vi "rotary_PKP214_stiffness_test.vi"() -> ()   [LabVIEW 2014]
uses:
  <vilib>/rvi/FXPMathLib/FxpSinAndCos/subVIs/nifxpmath_SinAndCos_SimConfig.ctl
  <vilib>/rvi/Emulation/niFpgaGetClockAttributes.vi
  <vilib>/rvi/Emulation/niFpgaSctlEmulationGetInTimedLoop.vi
  <vilib>/rvi/Emulation/niFpgaEmulationReportErrorSimple.vi
  <vilib>/rvi/eio/common/nirviEmuTemplateMethod_errors.vi
  <vilib>/rvi/Emulation/niFpgaProcessEmulError.vi
  <vilib>/rvi/Emulation/niFpgaCriticalErrorInLSC.vi
  <vilib>/rvi/FXPMathLib/FxpSinAndCos/simVIs/DllFxpSinAndCosTemp_sub.vi
  <vilib>/rvi/interface/RandomDataEmulation/nirviRandomDataMultiElementFPGAFIFO.vi
  <instcachedir>/0/nirviRandomDataMultiElementFPGAFIFO_AD0CFC12EF974623A9C2E4184BC062B2.lvgen/nirviRandomDataMultiElementFPGAFIFO_AD0CFC12EF974623A9C2E4184BC062B2_023.vi
  <vilib>/rvi/interface/RandomDataEmulation/niFpgaRandomDataHandleErrors.vi
  <vilib>/eio/EIONode/EIONode.xnode
  <vilib>/rvi/FXPMathLib/FxpMul/XNode/nifxpmath_Multiplier.xnode
  <vilib>/rvi/FXPMathLib/FxpSinAndCos/XNode/nifxpmath_SinAndCos.xnode
  <vilib>/rvi/Analysis/measure/butterworth/XNode/niFpgaButterworthFilter.xnode
  <vilib>/rvi/FXPMathLib/FxpSub/XNode/nifxpmath_Sub.xnode
  <vilib>/rvi/FXPMathLib/FxpAdd/XNode/nifxpmath_Add.xnode
  <vilib>/rvi/DataTransferAndStorage/Container/XNode/niFpgaContainer.xnode
  <vilib>/rvi/interface/RandomDataEmulation/nirviRandomDataFpgaMultiElementTemplate.vi
  <vilib>/rvi/FXPMathLib/sim/FxpSim.dll
panel:
  out "Thetamr_dd":fxp<+/-,36,29>
  in  "thetam_limit (rad)":fxp<+/-,22,8>
  in  "Load cell start":bool
  in  "Load cell stop":bool
  in  "Load cell reset":bool
  out "Load cell 0":fxp<+/-,60,14>
  out "Load cell 1":fxp<+/-,60,14>
  in  "Magnetic Encoder Reset":bool
  out "Magnetic Encoder Position":i32
  out "Theta_a":fxp<+/-,33,18>
  out "Thetam":fxp<+/-,33,18>
  in  "Frequency_start (Hz)":fxp<+/-,22,8>
  in  "Target time (s)":fxp<+/-,24,9>
  in  "Frequency_end (Hz)":fxp<+/-,23,8>
  out "Chirp_signal":fxp<+/-,36,11>
  in  "Sin wave ampitude (rad)":fxp<+/-,21,11>
  out "omega (M_avg)":fxp<+/-,64,35>
  in  "D_d_M_avg_Tc (uSec)":u32
  out "omega (M)":fxp<+/-,64,30>
  in  "D_d_M_Tc (uSec)":u32 format="%#_6f"
  out "omega(T)":fxp<+/-,20,9>
  in  "Velocity Estimation":i16(ring) items=["M_avg method", "M method", "T method"]
  out "Thetamr_ramp":fxp<+/-,64,30>
  out "Thetamr_slope":fxp<+/-,33,17>
  in  "Thetamr_time":fxp<+/-,16,11>
  out "Thetamr_sin":fxp<+/-,28,11>
  out "Thetamr_sin_d":fxp<+/-,64,16>
  out "Thetamr_sin_dd":fxp<+/-,64,25>
  out "Sin omega":fxp<+/-,41,8>
  in  "Sin offset":fxp<+/-,27,10>
  in  "Sin magnitude":fxp<+/-,17,8>
  in  "Sin wave frequency (Hz)":fxp<+/-,21,5>
  out "Time now (s)":fxp<+,52,14>
  out "Thetamr":fxp<+/-,64,31>
  in  "Thetamr_end":fxp<+/-,19,9>
  in  "Command type":i16(ring) items=["Step", "Ramp", "Sine", "Chirp"]
  out "Thetam_i":fxp<+/-,34,18>
  in  "D_tolorence":fxp<+/-,14,3>
  in  "Ki":fxp<+/-,22,9>
  out "Thetam_error":fxp<+/-,24,11>
  in  "Direction":bool
  out "taur":fxp<+/-,64,31>
  in  "Kd":fxp<+/-,20,8>
  in  "Kp":fxp<+/-,20,12>
  in  "scaled coefficients_D_dd":i32[](array[numeric])=[780119100, 146811362]
  out "Thetam_dd":fxp<+/-,36,29>
  in  "Ini coe.":bool
  out "va":fxp<+/-,38,8>
  out "vb":fxp<+/-,38,8>
  in  "stop motor":bool
  out "vq_F":fxp<+/-,20,5> format="%.57g"
  out "vd_F":fxp<+/-,20,5>
  out "mt":u32
  out "omega (rad/s)":fxp<+/-,32,18>
  in  "mt0":u32
  out "NrTheta":fxp<+/-,33,18>
  out "Encoder Position":i32
  in  "Encoder Reset":bool
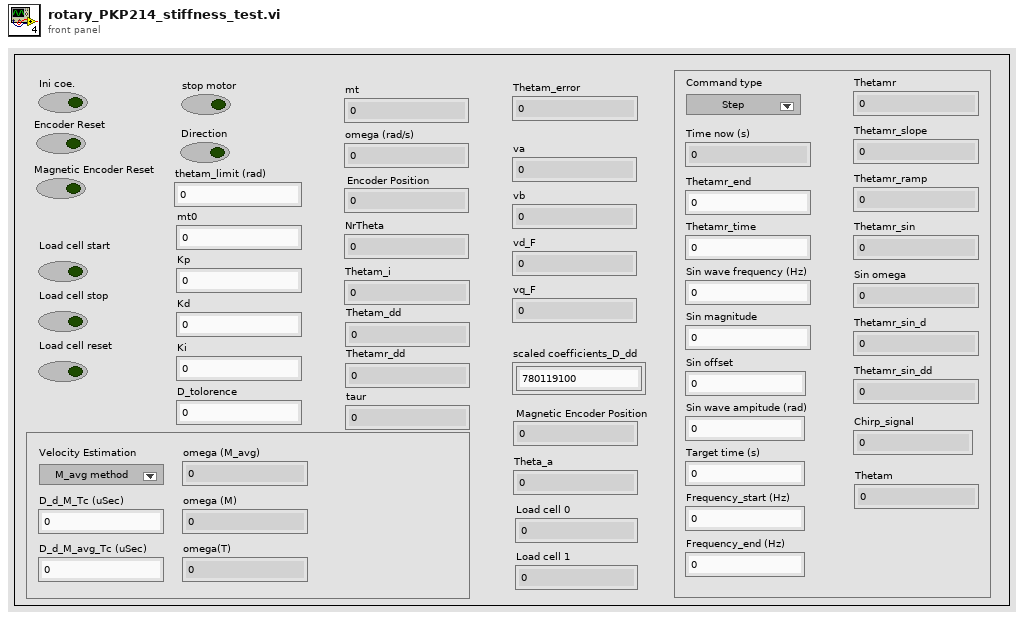
[diagram p1: front panel]
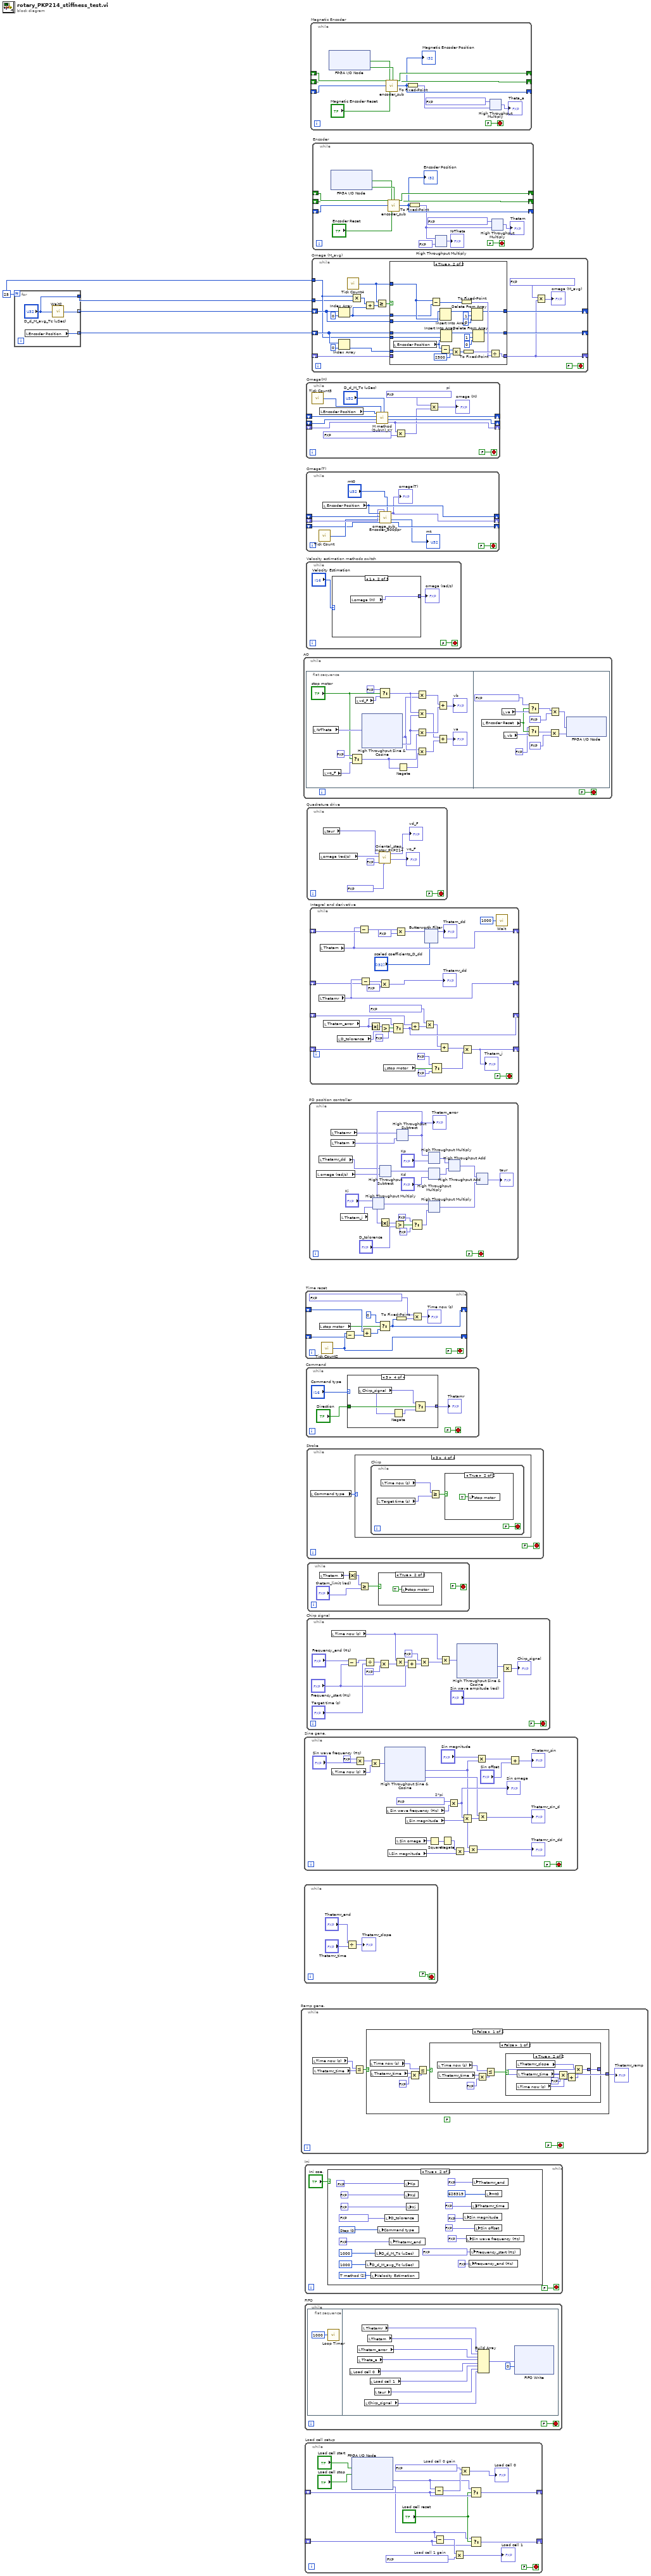
[diagram p0: block diagram]
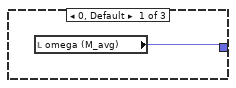
[diagram p4: hidden frame]
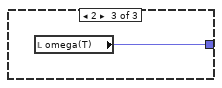
[diagram p5: hidden frame]
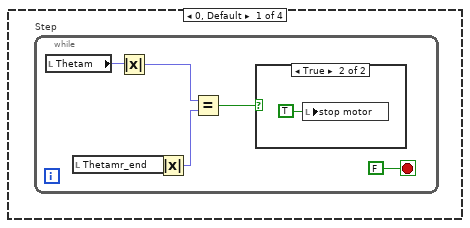
[diagram p6: hidden frame]
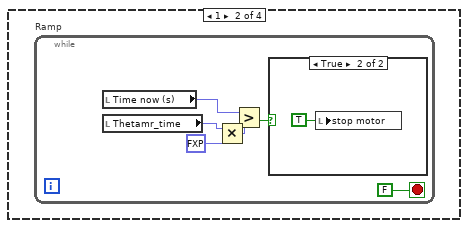
[diagram p8: hidden frame]
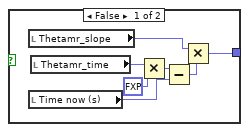
[diagram p12: hidden frame]
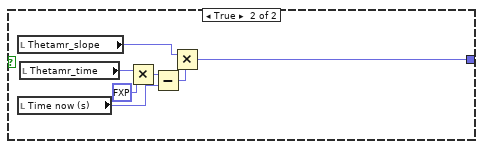
[diagram p13: hidden frame]
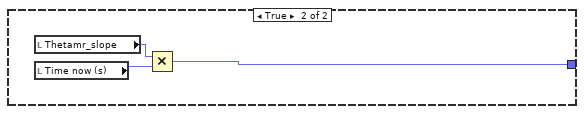
[diagram p14: hidden frame]
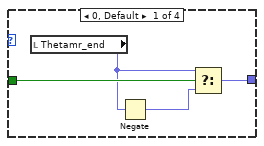
[diagram p15: hidden frame]
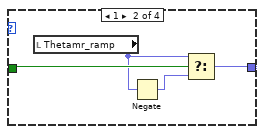
[diagram p16: hidden frame]
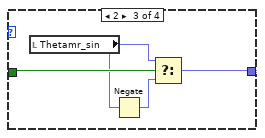
[diagram p17: hidden frame]
diagram:
  w4 = 25
  n1 = for {
    N: w4 -> [_]
    tunnel: ["D_d_M_avg_Tc (uSec)"] -> w1
    tunnel: [w6] -> w3 mode=indexing
    tunnel: [w5] -> w2 mode=indexing
    n2 = local read "Encoder Position"() -> (w5:i32)
    n3 = call "Wait2"("Count(uSec)"="D_d_M_avg_Tc (uSec)") -> ("Tick Count(uSec)"=w6:u32)
  }
  n4 = while "Ramp gene." {
    stop <- FALSE stop-if-true
    (unwired) FALSE
    n5 = local read "Time now (s)"() -> (w10:fxp<+,52,14>)
    n6 = local read "Thetamr_time"() -> (w11:fxp<+/-,16,11>)
    n7 = Less Or Equal?(x=w10, y=w11) -> (x <= y?=w9:bool)
    n8 = case shown="False" w9 {
      tunnel: [w13 w46] -> w8
      frame False {
        n9 = local read "Time now (s)"() -> (w18:fxp<+,52,14>)
        n10 = local read "Thetamr_time"() -> (w17:fxp<+/-,16,11>)
        n11 = Multiply(x=w17, y=fxp<+/-,24,9> 3.0) -> (x*y=w14:fxp<+/-,40,20>)
        n12 = Less Or Equal?(x=w18, y=w14) -> (x <= y?=w15:bool)
        n13 = case shown="False" w15 {
          tunnel: [w24 w44] -> w13
          frame False {
            n14 = local read "Time now (s)"() -> (w20:fxp<+,52,14>)
            n15 = local read "Thetamr_time"() -> (w21:fxp<+/-,16,11>)
            n16 = Multiply(x=w21, y=fxp<+/-,24,9> 5.0) -> (x*y=w23:fxp<+/-,40,20>)
            n17 = Less Or Equal?(x=w20, y=w23) -> (x <= y?=w19:bool)
            n18 = case shown="True" w19 {
              tunnel: [w25 w32] -> w24
              frame False {
                n19 = local read "Thetamr_slope"() -> (w26:fxp<+/-,33,17>)
                n20 = local read "Time now (s)"() -> (w30:fxp<+,52,14>)
                n21 = local read "Thetamr_time"() -> (w27:fxp<+/-,16,11>)
                n22 = Multiply(x=w27, y=fxp<+/-,24,9> 6.0) -> (x*y=w29:fxp<+/-,40,20>)
                n23 = Subtract(x=w29, y=w30) -> (x-y=w31:fxp<+/-,58,20>)
                n24 = Multiply(x=w26, y=w31) -> (x*y=w25:fxp<+/-,64,35>)
              }
              frame True {
                n25 = local read "Thetamr_slope"() -> (w33:fxp<+/-,33,17>)
                n26 = local read "Time now (s)"() -> (w37:fxp<+,52,14>)
                n27 = local read "Thetamr_time"() -> (w34:fxp<+/-,16,11>)
                n28 = Multiply(x=w34, y=fxp<+/-,24,9> -4.0) -> (x*y=w36:fxp<+/-,40,20>)
                n29 = Add(x=w36, y=w37) -> (x+y=w38:fxp<+/-,58,20>)
                n30 = Multiply(x=w33, y=w38) -> (x*y=w32:fxp<+/-,64,35>)
              }
            }
          }
          frame True {
            n31 = local read "Thetamr_slope"() -> (w39:fxp<+/-,33,17>)
            n32 = local read "Time now (s)"() -> (w43:fxp<+,52,14>)
            n33 = local read "Thetamr_time"() -> (w40:fxp<+/-,16,11>)
            n34 = Multiply(x=w40, y=fxp<+/-,24,9> 2.0) -> (x*y=w42:fxp<+/-,40,20>)
            n35 = Subtract(x=w42, y=w43) -> (x-y=w45:fxp<+/-,58,20>)
            n36 = Multiply(x=w39, y=w45) -> (x*y=w44:fxp<+/-,64,35>)
          }
        }
      }
      frame True {
        n37 = local read "Thetamr_slope"() -> (w48:fxp<+/-,33,17>)
        n38 = local read "Time now (s)"() -> (w47:fxp<+,52,14>)
        n39 = Multiply(x=w48, y=w47) -> (x*y=w46:fxp<+/-,64,30>)
      }
    }
    "Thetamr_ramp" <- w8
  }
  n40 = while "AO" {
    stop <- FALSE stop-if-true
    n41 = flat-sequence {
      frame #0 {
        n42 = local read "NrTheta"() -> (w65:fxp<+/-,33,18>)
        n43 = local read "vq_F"() -> (w63:fxp<+/-,20,5>)
        n44 = Select(t=fxp<+,20,5> 0.0, s="stop motor", f=w63) -> (s? t:f=w60:fxp<+/-,21,6>)
        n45 = local read "vd_F"() -> (w64:fxp<+/-,20,5>)
        n46 = xnode "High Throughput Sine & Cosine"("x (pi)"=w65) -> ("sin(x)"=w56:fxp<+/-,17,2>, "cos(x)"=w58:fxp<+/-,17,2>)
        n47 = Select(t=fxp<+,20,5> 0.0, s="stop motor", f=w64) -> (s? t:f=w57:fxp<+/-,21,6>)
        n48 = Negate(x=w60) -> (-x=w59:fxp<+/-,21,6>)
        n49 = Multiply(x=w57, y=w56) -> (x*y=w55:fxp<+/-,37,7>)
        n50 = Multiply(x=w57, y=w58) -> (x*y=w53:fxp<+/-,37,7>)
        n51 = Multiply(x=w58, y=w60) -> (x*y=w54:fxp<+/-,37,7>)
        n52 = Multiply(x=w56, y=w59) -> (x*y=w52:fxp<+/-,37,7>)
        n53 = Add(x=w55, y=w54) -> (x+y=→"vb":fxp<+/-,38,8>)
        n54 = Add(x=w53, y=w52) -> (x+y=→"va":fxp<+/-,38,8>)
      }
      frame #1 {
        n55 = local read "Encoder Reset"() -> (w99:bool)
        n56 = local read "va"() -> (w101:fxp<+/-,38,8>)
        n57 = local read "vb"() -> (w100:fxp<+/-,38,8>)
        n58 = Select(t=fxp<+/-,20,5> 3.899993896484375 ("y"), s=w99, f=w101) -> (s? t:f=w102:fxp<+/-,38,8>)
        n59 = Select(t=fxp<+/-,20,5> 0.0 ("y"), s=w99, f=w100) -> (s? t:f=w103:fxp<+/-,38,8>)
        n60 = Multiply(x=w103, y=fxp<+/-,20,5> -0.5) -> (x*y=w107:fxp<+/-,57,12>)
        n61 = Multiply(x=w102, y=fxp<+/-,20,5> -0.5) -> (x*y=w106:fxp<+/-,57,12>)
        n62 = xnode "FPGA I/O Node"("Mod8/AO0"=w106, "Mod8/AO1"=w107) -> ()  [unwired: 2 in, 2 out]
      }
    }
  }
  n63 = while {
    stop <- FALSE stop-if-true
    n64 = Divide(x="Thetamr_end", y="Thetamr_time") -> (x/y=→"Thetamr_slope":fxp<+/-,36,15>)
  }
  n65 = while "Sine gene." {
    stop <- FALSE stop-if-true
    w129 = fxp<+,20,3> 6.2831878662109375  # 2*pi
    n66 = local read "Time now (s)"() -> (w132:fxp<+,52,14>)
    n67 = Multiply(x=fxp<+,1,2> 2.0, y="Sin wave frequency (Hz)") -> (x*y=w133:fxp<+/-,21,6>)
    n68 = Multiply(x=w133, y=w132) -> (x*y=w113:fxp<+/-,64,20>)
    n69 = xnode "High Throughput Sine & Cosine"("x (pi)"=w113) -> ("sin(x)"=w117:fxp<+/-,16,2>, "cos(x)"=w124:fxp<+/-,16,2>)
    n70 = local read "Sin wave frequency (Hz)"() -> (w128:fxp<+/-,21,5>)
    n71 = local read "Sin magnitude"() -> (w119:fxp<+/-,17,8>)
    n72 = local read "Sin omega"() -> (w120:fxp<+/-,41,8>)
    n73 = local read "Sin magnitude"() -> (w123:fxp<+/-,17,8>)
    n74 = Square(x=w120) -> (x^2=w121:fxp<+,64,14>)
    n75 = Negate(x=w121) -> (-x=w118:fxp<+/-,64,15>)
    n76 = Multiply(x=w129, y=w128) -> (x*y=w125:fxp<+/-,41,8>)
    "Sin omega" <- w125
    n77 = Multiply(x=w118, y=w119) -> (x*y=w122:fxp<+/-,64,23>)
    n78 = Multiply(x=w125, y=w123) -> (x*y=w130:fxp<+/-,57,15>)
    n79 = Multiply(x=w117, y=w122) -> (x*y=→"Thetamr_sin_dd":fxp<+/-,64,25>)
    n80 = Multiply(x="Sin magnitude", y=w117) -> (x*y=w131:fxp<+/-,33,10>)
    n81 = Multiply(x=w124, y=w130) -> (x*y=→"Thetamr_sin_d":fxp<+/-,64,16>)
    n82 = Add(x=w131, y="Sin offset") -> (x+y=→"Thetamr_sin":fxp<+/-,34,11>)
  }
  n83 = while "Ini" {
    stop <- FALSE stop-if-true
    n84 = case shown="True" "Ini coe." {
      frame False {
      }
      frame True {
        w170 = i16 2 items=["M_avg method", "M method", "T method"] ("Velocity Estimation")
        w178 = i16 0 items=["Step", "Ramp", "Sine"] ("Command type")
        n85 = local write "D_d_M_avg_Tc (uSec)"(u32 1000 ("D_d_M_avg_Tc (uSec)")) -> ()
        n86 = local write "Velocity Estimation"(w170) -> ()
        n87 = local write "D_d_M_Tc (uSec)"(u32 1000 ("D_d_M_Tc (uSec)")) -> ()
        n88 = local write "Command type"(w178) -> ()
        n89 = local write "D_tolorence"(fxp<+/-,14,3> 0.009765625 ("D_tolorence")) -> ()
        n90 = local write "Thetamr_end"(fxp<+/-,16,11> 20.0 ("Dr_end")) -> ()
        n91 = local write "Kp"(fxp<+/-,20,12> 10.0 ("Kp")) -> ()
        n92 = local write "Kd"(fxp<+/-,20,8> 2.0 ("Kd")) -> ()
        n93 = local write "Ki"(fxp<+/-,20,6> 8.0 ("D_i")) -> ()
        n94 = local write "Sin magnitude"(fxp<+/-,11,8> 20.0 ("Sin magnitude")) -> ()
        n95 = local write "Sin wave frequency (Hz)"(fxp<+/-,21,5> 0.5 ("Sin wave frequency (Hz)")) -> ()
        n96 = local write "Frequency_end (Hz)"(fxp<+/-,23,8> 10.0 ("Frequency_end (Hz)")) -> ()
        n97 = local write "Frequency_start (Hz)"(fxp<+/-,20,5> 0.100006103515625 ("Frequency_start (Hz)")) -> ()
        n98 = local write "Thetamr_time"(fxp<+/-,16,11> 5.0 ("Dr_time")) -> ()
        n99 = local write "Thetamr_end"(fxp<+/-,11,7> 20.0 ("Fmr")) -> ()
        n100 = local write "Sin offset"(fxp<+/-,27,10> 0.0 ("Sin offset")) -> ()
        n101 = local write "mt0"(u32 628319 ("mt0")) -> ()
      }
    }
  }
  n102 = while "FIFO" {
    stop <- FALSE stop-if-true
    n103 = flat-sequence {
      frame #0 {
        n104 = call "Loop Timer"("Count(uSec)"=u32 1000) -> ()  [unwired: 1 out]
      }
      frame #1 {
        n105 = local read "Load cell 0"() -> (w187:fxp<+/-,60,14>)
        n106 = local read "Thetam_error"() -> (w192:fxp<+/-,24,11>)
        n107 = local read "Theta_a"() -> (w191:fxp<+/-,33,18>)
        n108 = local read "Thetamr"() -> (w194:fxp<+/-,64,31>)
        n109 = local read "Chirp_signal"() -> (w188:fxp<+/-,36,11>)
        n110 = local read "Thetam"() -> (w193:fxp<+/-,33,18>)
        n111 = local read "Load cell 1"() -> (w190:fxp<+/-,60,14>)
        n112 = local read "taur"() -> (w189:fxp<+/-,64,31>)
        n113 = Build Array(w194, w193, w192, w191, w187, w190, w189, w188) -> (w195:fxp<+/-,64,31>[])
        n114 = xnode ("FIFO Write")("Element"=w195, "Timeout"=0) -> ()  [unwired: 1 in, 2 out]
      }
    }
  }
  n115 = while "Load cell setup" {
    shift-right: [w209] -> _
    shift-left: _ -> [w206]
    shift-right: [w203] -> _
    shift-left: _ -> [w199]
    stop <- FALSE stop-if-true
    w198 = fxp<+/-,36,18> -10702.59870147705  # Load cell 0 gain
    w197 = fxp<+/-,36,18> -11003.09220123291  # Load cell 1 gain
    n116 = xnode "FPGA I/O Node"("Mod6/Start"="Load cell start", "Mod6/Stop"="Load cell stop") -> ("Mod6/AI3"=w207:fxp<+/-,24,-4>, "Mod6/AI2"=w200:fxp<+/-,24,-4>)  [unwired: 4 in, 4 out]
    n117 = Subtract(x=w207, y=w206) -> (x-y=w208:fxp<+/-,25,-3>)
    n118 = Subtract(x=w200, y=w199) -> (x-y=w201:fxp<+/-,25,-3>)
    n119 = Multiply(x=w201, y=w197) -> (x*y=→"Load cell 1":fxp<+/-,60,14>)
    n120 = Multiply(x=w198, y=w208) -> (x*y=→"Load cell 0":fxp<+/-,60,14>)
    n121 = Select(t=w207, s="Load cell reset", f=w206) -> (s? t:f=w209:fxp<+/-,24,-4>)
    n122 = Select(t=w200, s="Load cell reset", f=w199) -> (s? t:f=w203:fxp<+/-,24,-4>)
  }
  n123 = while "Time reset" {
    shift-right: [w216] -> _
    shift-left: _ -> [w223]
    shift-right: [w218] -> _
    shift-left: _ -> [w219]
    stop <- FALSE stop-if-true
    n124 = local read "stop motor"() -> (w221:bool)
    n125 = call "Tick Count2"() -> ("Tick Count(uSec)"=w218:u32)
    n126 = Subtract(x=w218, y=w219) -> (x-y=w224:u32)
    n127 = Add(x=w223, y=w224) -> (x+y=w222:u32)
    n128 = Select(t=u32 0, s=w221, f=w222) -> (s? t:f=w216:u32)
    n129 = To Fixed-Point(number=w216) -> (fixed-point=w215:fxp<+,32,32>)  [unwired: 1 in]
    n130 = Multiply(x=fxp<+,20,-18> 1.0000003385357559e-06, y=w215) -> (x*y=→"Time now (s)":fxp<+,52,14>)
  }
  n131 = while "Command" {
    stop <- FALSE stop-if-true
    n132 = case shown="3" "Command type" {
      tunnel: [w229 w233 w237 w241] -> w227
      tunnel: "Direction" -> [w232 w236 w240 w244]
      frame 0, Default {
        n133 = local read "Thetamr_end"() -> (w231:fxp<+/-,19,9>)
        n134 = Negate(x=w231) -> (-x=w230:fxp<+/-,20,10>)
        n135 = Select(t=w231, s=w232, f=w230) -> (s? t:f=w229:fxp<+/-,20,10>)
      }
      frame 1 {
        n136 = local read "Thetamr_ramp"() -> (w234:fxp<+/-,64,30>)
        n137 = Negate(x=w234) -> (-x=w235:fxp<+/-,64,31>)
        n138 = Select(t=w234, s=w236, f=w235) -> (s? t:f=w233:fxp<+/-,64,31>)
      }
      frame 2 {
        n139 = local read "Thetamr_sin"() -> (w238:fxp<+/-,28,11>)
        n140 = Negate(x=w238) -> (-x=w239:fxp<+/-,27,10>)
        n141 = Select(t=w238, s=w240, f=w239) -> (s? t:f=w237:fxp<+/-,28,11>)
      }
      frame 3 {
        n142 = local read "Chirp_signal"() -> (w242:fxp<+/-,36,11>)
        n143 = Negate(x=w242) -> (-x=w243:fxp<+/-,37,12>)
        n144 = Select(t=w242, s=w244, f=w243) -> (s? t:f=w241:fxp<+/-,37,12>)
      }
    }
    "Thetamr" <- w227
  }
  n145 = while "Omega(M)" {
    shift-right: [w256] -> _
    shift-left: _ -> [w257]
    shift-right: [w252] -> _
    shift-left: _ -> [w253]
    shift-right: [w250] -> _
    shift-left: _ -> [w251]
    stop <- FALSE stop-if-true
    w247 = fxp<+/-,27,3> 3.1415926218032837  # pi
    n146 = call "Tick Count3"() -> ("Tick Count(mSec)"=w255:u32)
    n147 = local read "Encoder Position"() -> (w258:i32)
    n148 = call "M method (SubVI)_KY.vi"("Tc (mSec)"="D_d_M_Tc (uSec)", "Tick Count (mSec)"=w255, "Encoder velocity_pre (pulse/s)"=w251, "Shift Register in 2"=w253, "Shift Register in 1"=w257, "Encoder pulses"=w258) -> ("Encoder velocity (pulse/s)"=w250:fxp<+/-,64,32>, "Shift Register out 2"=w252:i32, "Shift Register out 1"=w256:u32)  [unwired: 3 in]
    n149 = Multiply(x=w250, y=fxp<+/-,20,-5> 0.002499997615814209) -> (x*y=w248:fxp<+/-,64,27>)
    n150 = Multiply(x=w247, y=w248) -> (x*y=→"omega (M)":fxp<+/-,64,30>)
  }
  n151 = while "Omega(T)" {
    shift-right: [w267] -> _
    shift-left: _ -> [w268]
    shift-right: [w259] -> _
    shift-left: _ -> [w266]
    shift-right: [w263] -> _
    shift-left: _ -> [w264]
    stop <- FALSE stop-if-true
    n152 = call "Tick Count"() -> ("Tick Count(Ticks)"=w265:u32)
    n153 = local read "Encoder Position"() -> (w267:i32)
    n154 = call "omega_sub_Encoder_800ppr.vi"("mt0"="mt0", "omega_pre"=w266, "ticks_m_pre"=w264, "ticks"=w265, "count_pre"=w268, "count"=w267) -> ("ticks_m"=w263:u32, "mt"=→"mt":u32, "omega"=w259:fxp<+/-,20,9>)  [unwired: 3 in]
    "omega(T)" <- w259
  }
  n155 = while "Velocity estimation methods switch" {
    stop <- FALSE stop-if-true
    n156 = case shown="1" "Velocity Estimation" {
      tunnel: [w272 w273 w274] -> w270
      frame 0, Default {
        n157 = local read "omega (M_avg)"() -> (w272:fxp<+/-,64,35>)
      }
      frame 1 {
        n158 = local read "omega (M)"() -> (w273:fxp<+/-,64,30>)
      }
      frame 2 {
        n159 = local read "omega(T)"() -> (w274:fxp<+/-,20,9>)
      }
    }
    "omega (rad/s)" <- w270
  }
  n160 = while "Quadrature drive" {
    stop <- FALSE stop-if-true
    n161 = local read "omega (rad/s)"() -> (w279:fxp<+/-,32,18>)
    n162 = local read "taur"() -> (w280:fxp<+/-,64,31>)
    n163 = call "Oriental_step_motor_PKP214.vi"("tau_Threshold"=fxp<+,16,7> 0.00390625 ("F_Threshold"), "dtaumr"=fxp<+/-,25,15> 0.0 ("dFmr"), "omega"=w279, "taumr"=w280) -> ("vq_F"=→"vq_F":fxp<+/-,20,5>, "vd_F"=→"vd_F":fxp<+/-,20,5>)  [unwired: 6 in]
  }
  n164 = while "Stroke" {
    stop <- FALSE stop-if-true
    n165 = local read "Command type"() -> (w283:i16)
    n166 = case shown="3" w283 {
      frame 0, Default {
        n167 = while "Step" {
          stop <- FALSE stop-if-true
          n168 = local read "Thetam"() -> (w287:fxp<+/-,33,18>)
          n169 = local read "Thetamr_end"() -> (w289:fxp<+/-,19,9>)
          n170 = Absolute Value(x=w287) -> (abs(x)=w284:fxp<+,33,18>)
          n171 = Absolute Value(x=w289) -> (abs(x)=w288:fxp<+,19,9>)
          n172 = Equal?(x=w284, y=w288) -> (x = y?=w286:bool)
          n173 = case shown="True" w286 {
            frame False {
            }
            frame True {
              n174 = local write "stop motor"(TRUE ("stop motor")) -> ()
            }
          }
        }
      }
      frame 1 {
        n175 = while "Ramp" {
          stop <- FALSE stop-if-true
          n176 = local read "Time now (s)"() -> (w293:fxp<+,52,14>)
          n177 = local read "Thetamr_time"() -> (w295:fxp<+/-,16,11>)
          n178 = Multiply(x=w295, y=fxp<+/-,16,11> 6.0) -> (x*y=w292:fxp<+/-,32,22>)
          n179 = Greater?(x=w293, y=w292) -> (0:w291:bool)
          n180 = case shown="True" w291 {
            frame False {
            }
            frame True {
              n181 = local write "stop motor"(TRUE ("stop motor")) -> ()
            }
          }
        }
      }
      frame 2 {
      }
      frame 3 {
        n182 = while "Chirp" {
          stop <- FALSE stop-if-true
          n183 = local read "Target time (s)"() -> (w300:fxp<+/-,24,9>)
          n184 = local read "Time now (s)"() -> (w301:fxp<+,52,14>)
          n185 = Greater Or Equal?(x=w301, y=w300) -> (x >= y?=w299:bool)
          n186 = case shown="True" w299 {
            frame False {
            }
            frame True {
              n187 = local write "stop motor"(TRUE ("stop motor")) -> ()
            }
          }
        }
      }
    }
  }
  n188 = while "Chirp signal" {
    stop <- FALSE stop-if-true
    n189 = local read "Time now (s)"() -> (w311:fxp<+,52,14>)
    n190 = Subtract(x="Frequency_end (Hz)", y="Frequency_start (Hz)") -> (x-y=w303:fxp<+/-,24,9>)
    n191 = Divide(x=w303, y="Target time (s)") -> (x/y=w314:fxp<+/-,24,9>)
    n192 = Multiply(x=w314, y=fxp<+/-,24,9> 0.5) -> (x*y=w312:fxp<+/-,23,10>)
    n193 = Multiply(x=w311, y=w312) -> (x*y=w310:fxp<+/-,26,11>)
    n194 = Add(x=w310, y="Frequency_start (Hz)") -> (x+y=w309:fxp<+/-,22,8>)
    n195 = Multiply(x=fxp<+/-,3,3> 2.0, y=w309) -> (x*y=w307:fxp<+/-,25,10>)
    n196 = Multiply(x=w311, y=w307) -> (x*y=w316:fxp<+/-,33,18>)
    n197 = xnode "High Throughput Sine & Cosine"("x (pi)"=w316) -> ("sin(x)"=w319:fxp<+/-,16,2>)  [unwired: 1 out]
    n198 = Multiply(x=w319, y="Sin wave ampitude (rad)") -> (x*y=→"Chirp_signal":fxp<+/-,36,11>)
  }
  n199 = while {
    stop <- FALSE stop-if-true
    n200 = local read "Thetam"() -> (w351:fxp<+/-,33,18>)
    n201 = Absolute Value(x=w351) -> (abs(x)=w350:fxp<+,33,18>)
    n202 = Greater Or Equal?(x=w350, y="thetam_limit (rad)") -> (x >= y?=w353:bool)
    n203 = case shown="True" w353 {
      frame False {
      }
      frame True {
        n204 = local write "stop motor"(TRUE ("stop motor")) -> ()
      }
    }
  }
  n205 = while "PD position controller" {
    stop <- FALSE stop-if-true
    n206 = local read "omega (rad/s)"() -> (w357:fxp<+/-,32,18>)
    n207 = local read "Thetamr_dd"() -> (w356:fxp<+/-,36,29>)
    n208 = local read "Thetamr"() -> (w359:fxp<+/-,64,31>)
    n209 = local read "Thetam"() -> (w378:fxp<+/-,33,18>)
    n210 = local read "Thetam_i"() -> (w370:fxp<+/-,34,18>)
    n211 = xnode ("High Throughput Multiply")("x"="Ki", "y"=w370) -> ("x*y"=w364:fxp<+/-,56,27>)
    n212 = xnode "High Throughput Subtract"("x"=w356, "y"=w357) -> ("x-y"=w358:fxp<+/-,44,30>)
    n213 = xnode "High Throughput Subtract"("x"=w359, "y"=w378) -> ("x-y"=w368:fxp<+/-,64,32>)
    "Thetam_error" <- w368
    n214 = Absolute Value(x=w368) -> (abs(x)=w369:fxp<+,64,32>)
    n215 = Greater?(x=w369, y="D_tolorence") -> (0:w367:bool)
    n216 = Select(t=fxp<+,10,2> 1.0, s=w367, f=fxp<+,10,2> 0.0) -> (s? t:f=w363:fxp<+,10,2>)
    n217 = xnode ("High Throughput Multiply")("x"=w364, "y"=w363) -> ("x*y"=w360:fxp<+/-,64,29>)
    n218 = xnode ("High Throughput Multiply")("x"=w368, "y"="Kp") -> ("x*y"=w376:fxp<+/-,64,44>)
    n219 = xnode ("High Throughput Multiply")("x"=w358, "y"="Kd") -> ("x*y"=w375:fxp<+/-,64,38>)
    n220 = xnode ("High Throughput Add")("x"=w376, "y"=w375) -> ("x+y"=w361:fxp<+/-,64,45>)
    n221 = xnode ("High Throughput Add")("x"=w361, "y"=w360) -> ("x+y"=→"taur":fxp<+/-,64,46>)
  }
  n222 = while "Integral and derivative" {
    shift-right: [w404] -> _
    shift-left: _ -> [w408]
    shift-right: [w395] -> _
    shift-left: _ -> [w396]
    shift-right: [w385] -> _
    shift-left: _ -> [w389]
    shift-right: [w381] -> _
    shift-left: _ -> [w380]
    stop <- FALSE stop-if-true
    n223 = local read "Thetamr"() -> (w381:fxp<+/-,64,31>)
    n224 = local read "Thetam"() -> (w404:fxp<+/-,33,18>)
    n225 = local read "Thetam_error"() -> (w397:fxp<+/-,24,11>)
    n226 = local read "D_tolorence"() -> (w400:fxp<+/-,14,3>)
    n227 = Subtract(x=w404, y=w408) -> (x-y=w407:fxp<+/-,34,19>)
    n228 = Subtract(x=w381, y=w380) -> (x-y=w384:fxp<+/-,64,32>)
    n229 = Absolute Value(x=w397) -> (abs(x)=w401:fxp<+,24,11>)
    n230 = Multiply(x=w384, y=fxp<+/-,33,13> 1000.0) -> (x*y=→"Thetamr_dd":fxp<+/-,64,44>)
    n231 = Greater?(x=w401, y=w400) -> (0:w399:bool)
    n232 = local read "stop motor"() -> (w392:bool)
    n233 = Select(t=w397, s=w399, f=fxp<+,24,11> 0.0) -> (s? t:f=w395:fxp<+/-,25,12>)
    n234 = Multiply(x=w407, y=fxp<+/-,33,13> 1000.0) -> (x*y=w405:fxp<+/-,64,31>)
    n235 = Add(x=w396, y=w395) -> (x+y=w394:fxp<+/-,26,13>)
    n236 = Multiply(x=fxp<+/-,30,12> 0.000499725341796875, y=w394) -> (x*y=w388:fxp<+/-,55,24>)
    n237 = xnode "Butterworth Filter"("input data"=w405, "scaled coefficients"="scaled coefficients_D_dd") -> ("output data"=→"Thetam_dd":fxp<+/-,36,35>)  [unwired: 1 in]
    n238 = Select(t=fxp<+,1,1> 0.0, s=w392, f=fxp<+,1,1> 1.0) -> (s? t:f=w386:fxp<+,1,1>)
    n239 = Add(x=w388, y=w389) -> (x+y=w387:fxp<+/-,32,16>)
    n240 = Multiply(x=w387, y=w386) -> (x*y=w385:fxp<+/-,32,16>)
    "Thetam_i" <- w385
    n241 = call "Wait"("Count(uSec)"=u32 1000) -> ()  [unwired: 1 out]
  }
  n242 = while "Magnetic Encoder" {
    shift-right: [w425] -> _
    shift-left: _ -> [w427]
    shift-right: [w424] -> _
    shift-left: _ -> [w426]
    shift-right: [w422] -> _
    shift-left: _ -> [w423]
    stop <- FALSE stop-if-true
    n243 = xnode "FPGA I/O Node"() -> ("Mod7/DIO2"=w429:bool, "Mod7/DIO3"=w430:bool)  [unwired: 2 in, 2 out]
    n244 = call "encoder_sub.vi"("A_pre"=w427, "B_pre"=w426, "Encoder Position_pre"=w423, "A input"=w429, "Encoder Position Reset"="Magnetic Encoder Reset", "B input"=w430) -> ("A"=w425:bool, "B"=w424:bool, "Encoder Position (Counts)"=w422:i32)  [unwired: 19 in]
    "Magnetic Encoder Position" <- w422
    n245 = To Fixed-Point(number=w422) -> (fixed-point=w419:fxp<+/-,32,32>)  [unwired: 1 in]
    n246 = xnode ("High Throughput Multiply")("x"=fxp<+/-,24,0> 0.0015339851379394531 ("y"), "y"=w419) -> ("x*y"=→"Theta_a":fxp<+/-,56,32>)
  }
  n247 = while "Omega (M_avg)" {
    tunnel: w4 -> [w442]
    shift-right: [w435] -> _
    shift-left: w3 -> [w446]
    shift-right: [w434] -> _
    shift-left: _ -> [w437]
    shift-right: [w436] -> _
    shift-left: w2 -> [w445]
    tunnel: w1 -> [w439]
    stop <- FALSE stop-if-true
    n248 = Index Array(array=w446, index=0) -> (element=w440:u32)
    n249 = Index Array(array=w445, index=0) -> (element=w441:i32)
    n250 = call "Tick Count4"() -> ("Tick Count(uSec)"=w443:u32)
    n251 = Multiply(x=w442, y=w439) -> (x*y=w447:u32)
    n252 = Add(x=w447, y=w440) -> (x+y=w444:u32)
    n253 = Greater Or Equal?(x=w443, y=w444) -> (x >= y?=w438:bool)
    n254 = case shown="True" w438 {
      tunnel: w446 -> [w452 w469]
      tunnel: w445 -> [w451 w468]
      tunnel: w443 -> [_ w461]
      tunnel: w442 -> [_ w467]
      tunnel: w441 -> [_ w465]
      tunnel: w440 -> [_ w460]
      tunnel: w437 -> [w450 _]
      tunnel: [w451 w455] -> w436
      tunnel: [w452 w454] -> w435
      tunnel: [w450 w453] -> w434
      frame False {
      }
      frame True {
        n255 = local read "Encoder Position"() -> (w466:i32)
        n256 = Subtract(x=w461, y=w460) -> (x-y=w458:u32)
        n257 = Insert Into Array(array=w469, new element=w461) -> (w470:u32[])  [unwired: 1 in]
        n258 = Subtract(x=w466, y=w465) -> (x-y=w464:i32)
        n259 = Insert Into Array(array=w468, index=w467, new element=w466) -> (w471:i32[])
        n260 = Multiply(x=w464, y=2500) -> (x*y=w462:i32)
        n261 = To Fixed-Point(number=w458) -> (fixed-point=w456:fxp<+,32,32>)  [unwired: 1 in]
        n262 = To Fixed-Point(number=w462) -> (fixed-point=w457:fxp<+/-,32,32>)  [unwired: 1 in]
        n263 = Delete From Array(array=w470, length=1, index=0) -> (array with subset deleted=w454:u32[])  [unwired: 1 out]
        n264 = Delete From Array(array=w471, length=1, index=0) -> (array with subset deleted=w455:i32[])  [unwired: 1 out]
        n265 = Divide(x=w457, y=w456) -> (x/y=w453:fxp<+/-,64,32>)
      }
    }
    n266 = Multiply(x=fxp<+/-,27,3> 3.1415926218032837, y=w434) -> (x*y=→"omega (M_avg)":fxp<+/-,64,35>)
  }
  n267 = while "Encoder" {
    shift-right: [w483] -> _
    shift-left: _ -> [w485]
    shift-right: [w482] -> _
    shift-left: _ -> [w484]
    shift-right: [w480] -> _
    shift-left: _ -> [w481]
    stop <- FALSE stop-if-true
    n268 = xnode "FPGA I/O Node"() -> ("Mod7/DIO0"=w488:bool, "Mod7/DIO1"=w489:bool)  [unwired: 2 in, 2 out]
    n269 = call "encoder_sub.vi"("A_pre"=w485, "B_pre"=w484, "Encoder Position_pre"=w481, "A input"=w488, "Encoder Position Reset"="Encoder Reset", "B input"=w489) -> ("A"=w483:bool, "B"=w482:bool, "Encoder Position (Counts)"=w480:i32)  [unwired: 19 in]
    "Encoder Position" <- w480
    n270 = To Fixed-Point(number=w480) -> (fixed-point=w476:fxp<+/-,32,32>)  [unwired: 1 in]
    n271 = xnode ("High Throughput Multiply")("x"=w476, "y"=fxp<+/-,24,0> 0.125) -> ("x*y"=→"NrTheta":fxp<+/-,56,32>)
    n272 = xnode ("High Throughput Multiply")("x"=fxp<+/-,24,0> 0.007853984832763672 ("y"), "y"=w476) -> ("x*y"=→"Thetam":fxp<+/-,56,32>)
  }
